vi "Test Find Chessboard Corners Sector Based.vi"(8 "error in (no error)":errorcluster, 11 "Test Case In":refnum<class "02_FeatureDetection.lvclass">) -> (0 "error out":errorcluster, 3 "Test Case Out":refnum<class "02_FeatureDetection.lvclass">)   [LabVIEW 2020, in "test.lvlib" / "02_FeatureDetection.lvclass"]
uses:
  02_FeatureDetection.lvclass
  C:/Program Files (x86)/National Instruments/LabVIEW 2026/vi.lib/Astemes/LUnit/Test Case.lvclass
  ar/Find Chessboard Corners Sector Based Flags.ctl
  common/Image Size (Integer).ctl
  ar/Chessboard Corner Info.ctl
  common/Image Point (Float).ctl
  <vilib>/Astemes/LUnit/Test Case.lvclass/Test Case.ctl
  image/Line Type.ctl
  image/New Image (Greyscale Array).vi
  ar/Find Chessboard Corners (Greyscale Sector Based).vi
  image/Draw Circle (Greyscale).vi
  image/Draw Rectangle (Greyscale).vi
  image/Draw Image to Picture (Greyscale).vi
  ar/DrawChessboardSemiCircleSquare.vi
  ar/DrawChessboardTearDropSquare.vi
  ar/DrawChessboardSpotOnSquare.vi
  ar/Generate Chessboard Image Data (Radon).vi/e7f4303d-582b-4721-b29a-aa63d9231187.vi
  common/PictureToGreyscaleArrayData.vi
  ar/Find Chessboard Corners (Greyscale Sector Based).vi/6a9761e7-0504-45a6-89a0-1e961674e9fc.vi
  <vilib>/Astemes/LUnit/Core/LUnit Test Case/Private/Append Fail Result.vi
  <vilib>/Astemes/LUnit/Core/LUnit Test Case/Private/Append Pass Result.vi
  image/Draw Circle (Greyscale).vi/8336a1cf-e433-4bea-8080-376bdb783d4e.vi
  image/Draw Rectangle (Greyscale).vi/7e6fb015-3761-4366-a0a7-e436eb229083.vi
  image/Draw Image to Picture (Greyscale).vi/9ae995ca-ccda-485c-89ac-02736fde3e8e.vi
  <vilib>/Astemes/LUnit/Core/LUnit Test Case/Private/Run In UI.vi
  <vilib>/Utility/error.llb/Clear Errors.vi
  <vilib>/picture/picture.llb/Draw Oval.vi
  <vilib>/picture/picture.llb/Draw Rectangle.vi
  <vilib>/picture/pictutil.llb/Picture to Pixmap.vi
  <vilib>/picture/pixmap.llb/Unflatten Pixmap.vi
  <vilib>/Utility/error.llb/Error Cluster From Error Code.vi
  <vilib>/Comparison/Equal/Equal Functor/Equal Functor.lvclass
  image/image.lvlib
  ar/ar.lvlib
  <vilib>/Astemes/LUnit/Test Case.lvclass
  common/common.lvlib
panel:
  out "Picture":picture
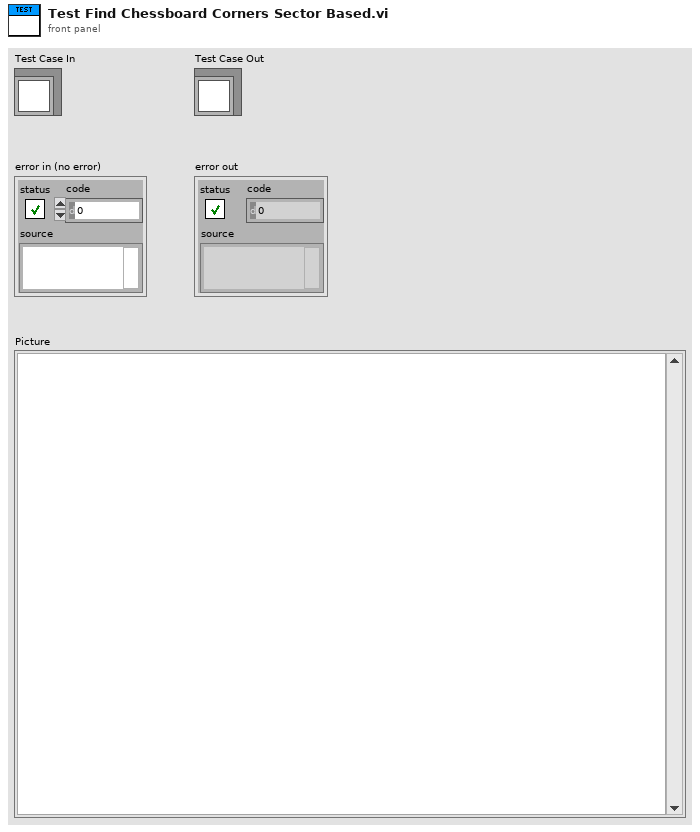
[diagram p1: front panel]
types:
  T1 = typedef "common.lvlib/Image Point (Float).ctl" = cluster{"x":dbl, "y":dbl}
  T2 = typedef "ar.lvlib/Chessboard Corner Info.ctl" = cluster{"Points Per Row":u8, "Points Per Col":u8}
  T3 = typedef "common.lvlib/Image Size (Integer).ctl" = cluster{"Width":u16, "Height":u16}
  T4 = typedef "ar.lvlib/Find Chessboard Corners Sector Based Flags.ctl" = enum16{"CALIB_CB_NORMALIZE_IMAGE", "CALIB_CB_EXHAUSTIVE", "CALIB_CB_ACCURACY", "CALIB_CB_LARGER", "CALIB_CB_MARKER"}
  T5 = typedef "image.lvlib/Greyscale Image.ctl" = refnum<data-value>
  T6 = typedef "ar.lvlib/Find Chessboard Corners Sector Based Meta.ctl" = enum16{"No Meta Data", "Left-Top Corner Black Cell", "Left-Top Corner White Cell", "Left-Top Corner Black Cell with Marker", "Left-Top Corner White Cell with Marker"}
  T7 = typedef "image.lvlib/Line Type.ctl" = enum8{"FILLED", "LINE_4", "LINE_8", "LINE_AA"}
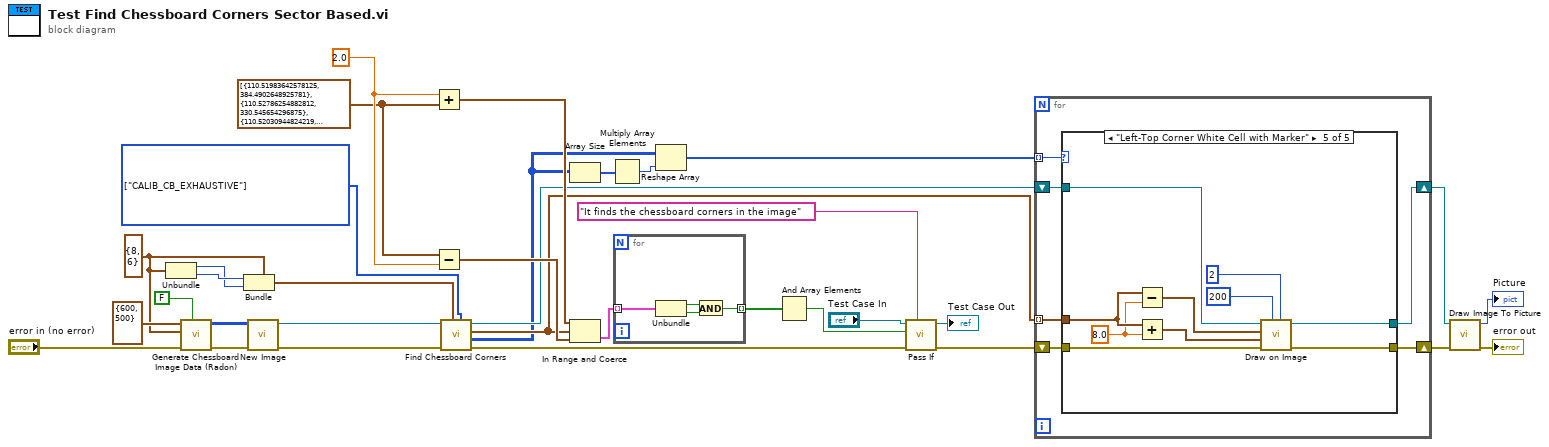
[diagram p0: block diagram]
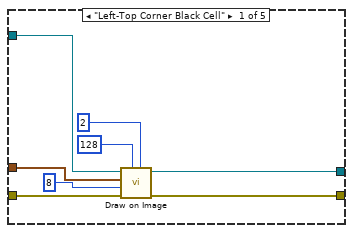
[diagram p2: hidden frame]
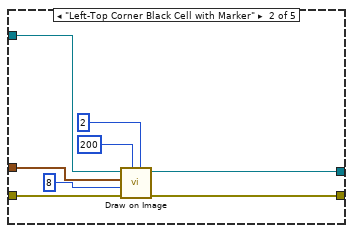
[diagram p3: hidden frame]
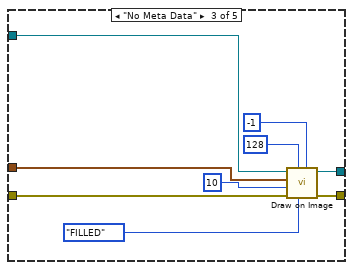
[diagram p4: hidden frame]
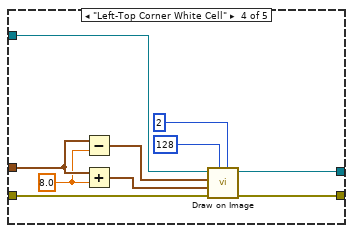
[diagram p5: hidden frame]
diagram:
  w4 = T1[] [{"x"=110.51983642578125, "y"=384.4902648925781}, {"x"=110.52786254882812, "y"=330.545654296875}, {"x"=110.52030944824219, "y"=276.5110168457031}, {"x"=110.52304077148438, "y"=222.49684143066406}, {"x"=110.52587127685547, "y"=168.5770263671875}, {"x"=110.5278549194336, "y"=114.48518371582031}, {"x"=164.4899139404297, "y"=384.4825744628906}, {"x"=164.49302673339844, "y"=330.5461730957031}, {"x"=164.4706268310547, "y"=276.5264892578125}, {"x"=164.47882080078125, "y"=222.49041748046875}, {"x"=164.487060546875, "y"=168.57138061523438}, {"x"=164.49017333984375, "y"=114.49085235595703}, {"x"=218.58425903320312, "y"=384.4807434082031}, {"x"=218.58438110351562, "y"=330.5576477050781}, {"x"=218.56167602539062, "y"=276.5283508300781}, {"x"=218.5755615234375, "y"=222.49874877929688}, {"x"=218.56430053710938, "y"=168.5651092529297}, {"x"=218.57057189941406, "y"=114.4876708984375}, {"x"=272.4980773925781, "y"=384.4714050292969}, {"x"=272.4951477050781, "y"=330.5459289550781}, {"x"=272.4820861816406, "y"=276.52618408203125}, {"x"=272.4815368652344, "y"=222.4823455810547}, {"x"=272.4978942871094, "y"=168.5762939453125}, {"x"=272.4895324707031, "y"=114.4795150756836}, {"x"=326.50860595703125, "y"=384.4912109375}, {"x"=326.507568359375, "y"=330.5517578125}, {"x"=326.52020263671875, "y"=276.52099609375}, {"x"=326.5254211425781, "y"=222.48287963867188}, {"x"=326.52752685546875, "y"=168.56243896484375}, {"x"=326.525634765625, "y"=114.47119903564453}, {"x"=380.5481262207031, "y"=384.49346923828125}, {"x"=380.5423278808594, "y"=330.5431213378906}, {"x"=380.5509948730469, "y"=276.5083312988281}, {"x"=380.5451354980469, "y"=222.4959716796875}, {"x"=380.55682373046875, "y"=168.58506774902344}, {"x"=380.54541015625, "y"=114.49372100830078}, {"x"=434.4837646484375, "y"=384.4846496582031}, {"x"=434.4927062988281, "y"=330.54888916015625}, {"x"=434.49041748046875, "y"=276.5093688964844}, {"x"=434.4705810546875, "y"=222.49887084960938}, {"x"=434.4798889160156, "y"=168.5850067138672}, {"x"=434.4817810058594, "y"=114.49042510986328}, {"x"=488.5366516113281, "y"=384.4859619140625}, {"x"=488.5210876464844, "y"=330.5379638671875}, {"x"=488.5309143066406, "y"=276.51507568359375}, {"x"=488.5359191894531, "y"=222.48826599121094}, {"x"=488.5423278808594, "y"=168.5687713623047}, {"x"=488.54949951171875, "y"=114.49140167236328}] ("Points")
  w12 = T2 {"Points Per Row"=8, "Points Per Col"=6} ("Chessboard Corners Info")
  w3 = T4[] [enum."CALIB_CB_EXHAUSTIVE"] items=["CALIB_CB_NORMALIZE_IMAGE", "CALIB_CB_EXHAUSTIVE", "CALIB_CB_ACCURACY", "CALIB_CB_LARGER", "CALIB_CB_MARKER"] ("Flags (Default: None)")
  w34 = 2.0
  n1 = Unbundle(w12) -> ("Points Per Row"=w10:u8, "Points Per Col"=w11:u8)
  n2 = call "Generate Chessboard Image Data (Radon).vi"("Add Marker (Default: False)"=FALSE, "error in (no error)"="error in (no error)", "Chessboard Corners Info"=w12, "Target Size"=T3 {"Width"=600, "Height"=500}) -> ("error out"=w21:errorcluster, "Chessboard Image Data"=w1:u8[][])  [unwired: 6 in]
  n3 = Bundle(cluster=w12, "Points Per Row"=w11, "Points Per Col"=w10) -> (w2:T2)
  n4 = call-poly "New Image.vi"("error in (no error)"=w21, "U8 Greyscale Data"=w1) -> ("error out"=w20:errorcluster, "Greyscale Image"=w19:T5)  [unwired: 8 in]
  n5 = Add(x=w34, y=w4) -> (x+y=w29:T1[])
  n6 = Subtract(x=w4, y=w34) -> (x-y=w30:T1[])
  n7 = call-poly "Find Chessboard Corners.vi"("Flags (Default: None)"=w3, "Chessboard Corners Info"=w2, "error in (no error)"=w20, "Greyscale Image in"=w19) -> ("error out"=w33:errorcluster, "Meta Data"=w8:T6[][], "Points"=w9:T1[], "Greyscale Image"=w17:T5)  [unwired: 4 in]
  n8 = Array Size(array=w8) -> (size(s)=w7:i32[])
  n9 = In Range and Coerce(upper limit=w29, x=w9, lower limit=w30) -> (In Range?=w28:cluster{"x":bool, "y":bool}[])  [unwired: 1 out]
  n10 = Multiply Array Elements(1:w7) -> (0:w6:i32)
  n11 = for {
    tunnel: w28 -> [w38] mode=indexing
    tunnel: [w35] -> w27 mode=indexing
    n12 = Unbundle(w38) -> ("x"=w37:bool, "y"=w36:bool)
    n13 = And(x=w37, y=w36) -> (x .and. y?=w35:bool)
  }
  n14 = Reshape Array(w8, w6) -> (w5:T6[])
  n15 = And Array Elements(Boolean array=w27) -> (logical AND=w26:bool)
  n16 = call <vilib>:"Pass If.vi"("Description"="It finds the chessboard corners in the image", "error in (no error)"=w33, "Pass?"=w26, "LUnit Test Case In"="Test Case In") -> ("error out"=w15:errorcluster, "LUnit Test Case Out"=→"Test Case Out":refnum<class "02_FeatureDetection.lvclass">)  [unwired: 6 in]
  n17 = for {
    shift-right: [w41] -> w16
    shift-left: w17 -> [w44]
    shift-right: [w42] -> w14
    shift-left: w15 -> [w43]
    tunnel: w9 -> [w40] mode=indexing
    tunnel: w5 -> [w39] mode=indexing
    n18 = case shown="\"Left-Top Corner White Cell with Marker\"" w39 {
      tunnel: w44 -> [w52 w60 w69 w79 w89]
      tunnel: w43 -> [w51 w59 w68 w78 w88]
      tunnel: [w50 w58 w67 w77 w87] -> w42
      tunnel: [w49 w57 w66 w76 w86] -> w41
      tunnel: w40 -> [w48 w56 w65 w74 w84]
      frame "Left-Top Corner Black Cell" {
        n19 = call-poly "Draw on Image.vi"("Thickness (Default: 1)"=2, "Colour"=u8 128, "error in (no error)"=w51, "Radius"=u16 8, "Centre"=w48, "Greyscale Image in"=w52) -> ("error out"=w50:errorcluster, "Greyscale Image"=w49:T5)  [unwired: 4 in]
      }
      frame "Left-Top Corner Black Cell with Marker" {
        n20 = call-poly "Draw on Image.vi"("Thickness (Default: 1)"=2, "Colour"=u8 200, "error in (no error)"=w59, "Radius"=u16 8, "Centre"=w56, "Greyscale Image in"=w60) -> ("error out"=w58:errorcluster, "Greyscale Image"=w57:T5)  [unwired: 4 in]
      }
      frame "No Meta Data" {
        n21 = call-poly "Draw on Image.vi"("Thickness (Default: 1)"=-1, "OpenCV Line Type (Default LINE_8)"=Line_Type."FILLED", "Colour"=u8 128, "error in (no error)"=w68, "Radius"=u16 10, "Centre"=w65, "Greyscale Image in"=w69) -> ("error out"=w67:errorcluster, "Greyscale Image"=w66:T5)  [unwired: 3 in]
      }
      frame "Left-Top Corner White Cell" {
        w73 = 8.0
        n22 = Subtract(x=w74, y=w73) -> (x-y=w75:T1)
        n23 = Add(x=w74, y=w73) -> (x+y=w72:T1)
        n24 = call-poly "Draw on Image.vi"("Thickness (Default: 1)"=2, "Colour"=u8 128, "error in (no error)"=w78, "Point B"=w72, "Point A"=w75, "Greyscale Image in"=w79) -> ("error out"=w77:errorcluster, "Greyscale Image"=w76:T5)  [unwired: 4 in]
      }
      frame "Left-Top Corner White Cell with Marker" {
        w83 = 8.0
        n25 = Subtract(x=w84, y=w83) -> (x-y=w85:T1)
        n26 = Add(x=w84, y=w83) -> (x+y=w82:T1)
        n27 = call-poly "Draw on Image.vi"("Thickness (Default: 1)"=2, "Colour"=u8 200, "error in (no error)"=w88, "Point B"=w82, "Point A"=w85, "Greyscale Image in"=w89) -> ("error out"=w87:errorcluster, "Greyscale Image"=w86:T5)  [unwired: 4 in]
      }
    }
  }
  n28 = call-poly "Draw Image To Picture.vi"("error in (no error)"=w14, "Greyscale Image Source in"=w16) -> ("error out"=→"error out":errorcluster, "Picture"=→"Picture":picture)  [unwired: 8 in]
